vi "Remove Extra Spaces.vi"(8 "error in (no error)":errorcluster, 10 "Input":string, 11 "Tovey 9150 in":refnum<class "Tovey 9150.lvclass">) -> (0 "error out":errorcluster, 2 "Output":string, 3 "Tovey 9150 out":refnum<class "Tovey 9150.lvclass">)   [LabVIEW 2015, in "Tovey 9150.lvclass"]
uses:
  Tovey 9150.lvclass
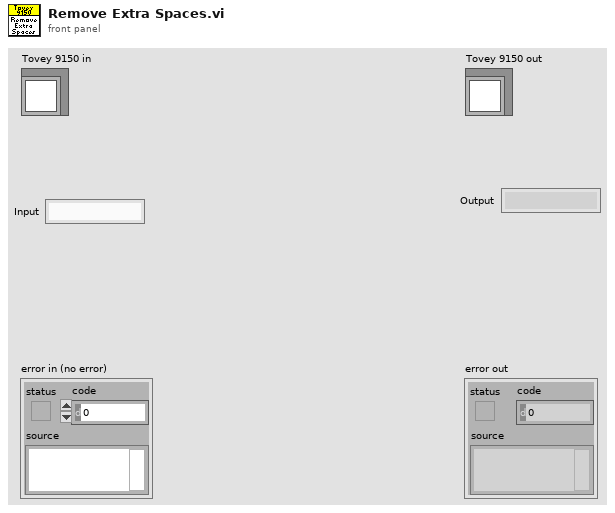
[diagram p1: front panel]
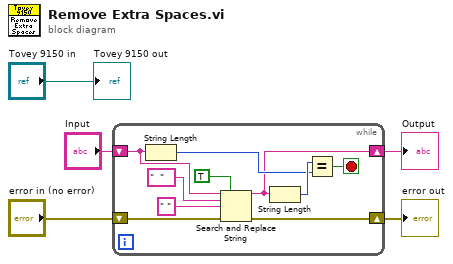
[diagram p0: block diagram]
diagram:
  n1 = while {
    shift-right: [w10] -> w3
    shift-left: "Input" -> [w12]
    shift-right: [w7] -> w1
    shift-left: "error in (no error)" -> [w8]
    stop <- w13 stop-if-true
    n2 = String Length(string=w12) -> (length=w14:i32)
    n3 = Search and Replace String(replace all?=TRUE ("replace all? (F)"), input string=w12, search string="  " ("substring (\"\")"), replace string=" " ("replace string (\"\")"), error in=w8) -> (result string=w10:string, error out=w7:errorcluster)  [unwired: 3 in, 2 out]
    n4 = String Length(string=w10) -> (length=w15:i32)
    n5 = Equal?(x=w15, y=w14) -> (x = y?=w13:bool)
  }
  "error out" <- w1
  "Output" <- w3
  "Tovey 9150 out" <- "Tovey 9150 in"
